vi "Abort Sequence-Load Ganging.vi"(8 "error in":errorcluster, 11 "Abort Sequence - Ganging":T1) -> (0 "error out":errorcluster)   [LabVIEW 2021]
doc: "Abort the sequence and if error resets the device for ganging configuration."
uses:
  controls/Abort Sequence-Ganging.ctl
  channel ganging/shared subVIs/ctl/NIDCPower_channel_ganging - ctl - ganged config.ctl
  channel ganging/shared subVIs/ctl/NIDCPower_channel_ganging - ctl - channel mode.ctl
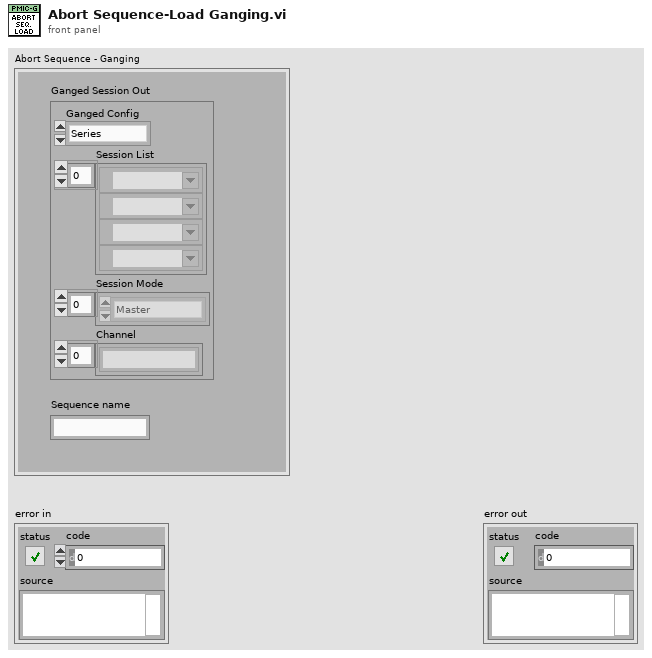
[diagram p1: front panel]
types:
  T1 = typedef "Abort Sequence-Ganging.ctl" = cluster{"Ganged Session Out":cluster{"Ganged Config":T2, "Session List":refnum<k15>[], "Session Mode":T3[], "Channel":string[]}, "Sequence name":string}
  T2 = typedef "NIDCPower_channel_ganging - ctl - ganged config.ctl" = enum32{"Series", "Parallel", "Manual"}
  T3 = typedef "NIDCPower_channel_ganging - ctl - channel mode.ctl" = enum32{"Master", "Slave", "Slave - Inverted"}
  T4 = cluster{"Ganged Config":T2, "Session List":refnum<k15>[], "Session Mode":T3[], "Channel":string[]}
  T5 = typedef "NIDCPower_channel_ganging - ctl - ganged session.ctl" = cluster{"Ganged Config":T2, "Session List":refnum<k15>[], "Session Mode":T3[], "Channel":string[]}
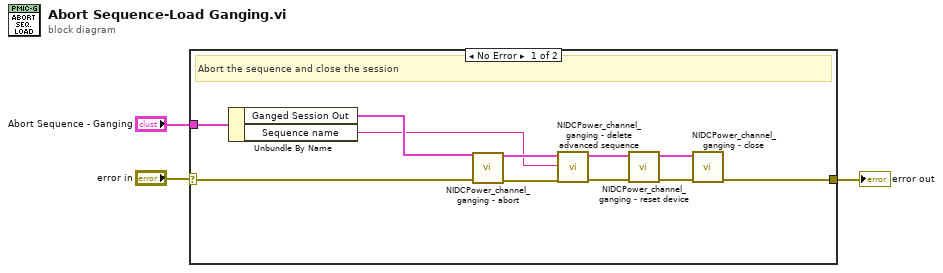
[diagram p0: block diagram]
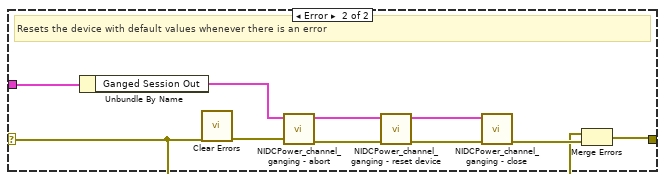
[diagram p2: hidden frame]
diagram:
  n1 = case shown="No Error" "error in" {
    selector: "error in" -> [w10 w16]
    tunnel: "Abort Sequence - Ganging" -> [w14 w24]
    tunnel: [w11 w15] -> w2
    frame No Error {
      # "Abort the sequence and close the session"
      n2 = Unbundle By Name(w14) -> ("Ganged Session Out"=w13:T4, "Sequence name"=w8:string)
      n3 = call "NIDCPower_channel_ganging - abort.vi"("error in (no error)"=w10, "Ganged Session In"=w13) -> ("error out"=w9:errorcluster, "Ganged Session Out"=w12:T5)  [unwired: 8 in]
      n4 = call "NIDCPower_channel_ganging - delete advanced sequence.vi"("error in (no error)"=w9, "sequence name"=w8, "Ganged Session In"=w12) -> ("error out"=w7:errorcluster, "Ganged Session Out"=w4:T5)  [unwired: 7 in]
      n5 = call "NIDCPower_channel_ganging - reset device.vi"("error in (no error)"=w7, "Ganged Session In"=w4) -> ("error out"=w6:errorcluster, "Ganged Session Out"=w5:T5)  [unwired: 8 in]
      n6 = call "NIDCPower_channel_ganging - close.vi"("error in (no error)"=w6, "Ganged Session In"=w5) -> ("error out"=w11:errorcluster)  [unwired: 9 in]
    }
    frame Error {
      # "Resets the device with default values whenever there is an error"
      n7 = Unbundle By Name(w24) -> ("Ganged Session Out"=w19:T4)
      n8 = call <vilib>:"Clear Errors.vi"("error in (no error)"=w16) -> ("error out"=w18:errorcluster)  [unwired: 5 in, 1 out]
      n9 = call "NIDCPower_channel_ganging - abort.vi"("error in (no error)"=w18, "Ganged Session In"=w19) -> ("error out"=w22:errorcluster, "Ganged Session Out"=w23:T5)  [unwired: 8 in]
      n10 = call "NIDCPower_channel_ganging - reset device.vi"("error in (no error)"=w22, "Ganged Session In"=w23) -> ("error out"=w20:errorcluster, "Ganged Session Out"=w21:T5)  [unwired: 8 in]
      n11 = call "NIDCPower_channel_ganging - close.vi"("error in (no error)"=w20, "Ganged Session In"=w21) -> ("error out"=w17:errorcluster)  [unwired: 9 in]
      n12 = Merge Errors(w16, w17) -> (w15:errorcluster)
    }
  }
  "error out" <- w2
